vi "Simulated_AnalogInput.vi"(8 "error in (no error)":errorcluster, 11 "Device Name":tag) -> (0 "error out":errorcluster, 3 "data":dynamicdata(waveform))   [LabVIEW 2023]
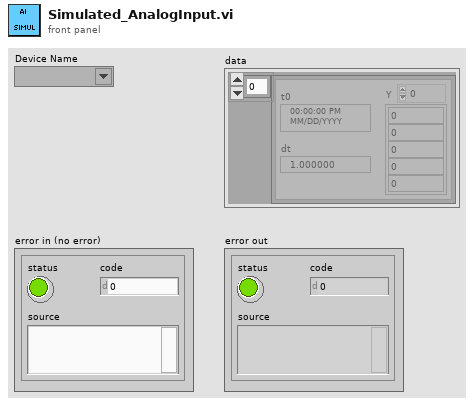
[diagram p1: front panel]
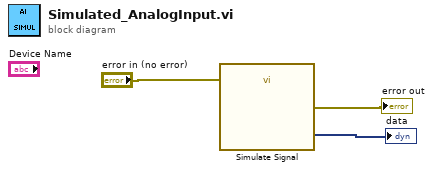
[diagram p0: block diagram]
diagram:
  n1 = call "Simulate Signal"("error in (no error)"="error in (no error)") -> ("DC with Uniform Noise"=→"data":dynamicdata, "error out"=→"error out":errorcluster)  [unwired: 13 in]
